vi "Load_Source_Type.vi"(8 "error in (no error)":errorcluster, 9 "index":i32, 11 "buildObject":T1) -> (0 "error out":errorcluster, 3 "AB_Source out":refnum<class "AB_Source.lvclass">)   [LabVIEW 2020, in "AB_Source.lvclass"]
uses:
  <vilib>/AppBuilder/AB_Classes/Source/AB_Source.lvclass
  <resource>/Framework/Providers/API/ItemRef.ctl
  <vilib>/AppBuilder/AB_Classes/Source/VI/AB_Source_VI.lvclass
  e:/builds/penguin/labview/branches/2020/dev/dist/vi.lib/AppBuilder/AB_Classes/Source/AB_Source.lvclass
  <vilib>/AppBuilder/AB_Classes/Source/ExportedVI/AB_Source_ExportedVI.lvclass
  <vilib>/AppBuilder/AB_Classes/Source/RESTfulVI/AB_Source_RESTfulVI.lvclass
  <vilib>/AppBuilder/AB_Classes/Source/Container/AB_Source_Container.lvclass
  <vilib>/AppBuilder/AB_Classes/Source/Library/AB_Source_Library.lvclass
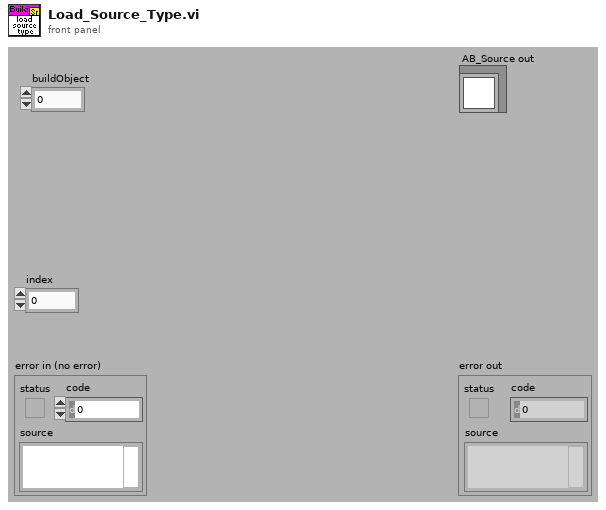
[diagram p1: front panel]
types:
  T1 = typedef "ItemRef.ctl" = u64
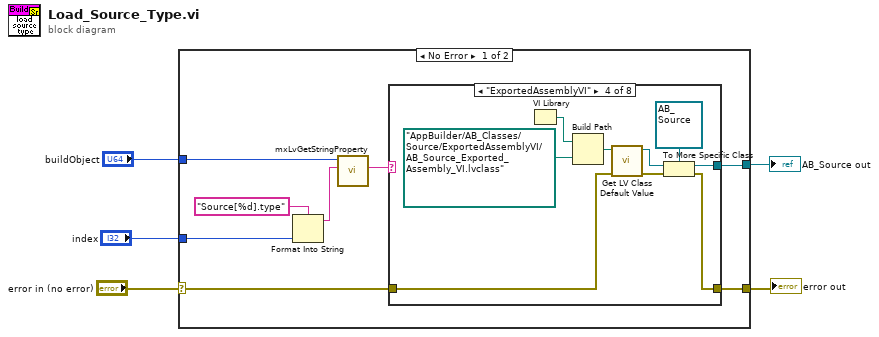
[diagram p0: block diagram]
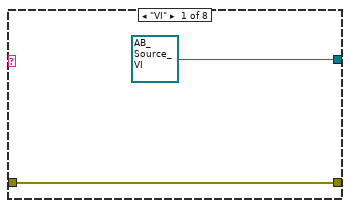
[diagram p2: hidden frame]
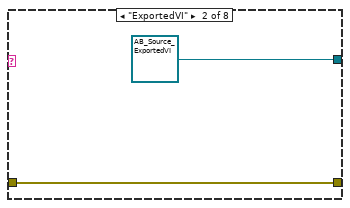
[diagram p3: hidden frame]
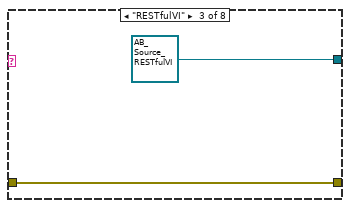
[diagram p4: hidden frame]
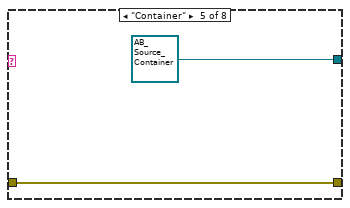
[diagram p5: hidden frame]
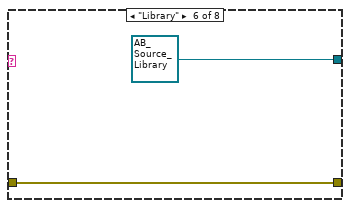
[diagram p6: hidden frame]
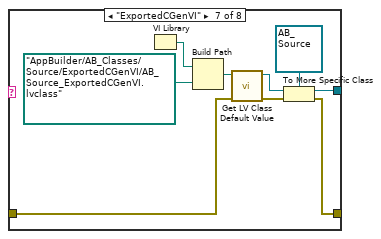
[diagram p7: hidden frame]
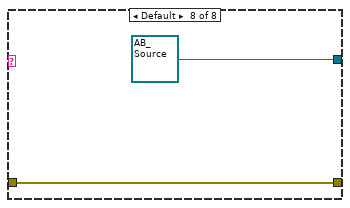
[diagram p8: hidden frame]
diagram:
  n1 = case shown="No Error" "error in (no error)" {
    selector: "error in (no error)" -> [w7 w44]
    tunnel: [w6 w44] -> w4
    tunnel: [w8 _] -> w3
    tunnel: "buildObject" -> [w13 _]
    tunnel: "index" -> [w10 _]
    frame No Error {
      n2 = Format Into String(format string="Source[%d].type", w10) -> (resulting string=w11:string)  [unwired: 2 in, 1 out]
      n3 = call <resource>:"mxLvGetStringProperty.vi"("Tag"=w11, "Item"=w13) -> ("Value"=w9:string)  [unwired: 1 in, 8 out]
      n4 = case shown="\"ExportedAssemblyVI\"" w9 {
        tunnel: [refnum<class "AB_Source_VI.lvclass"> refnum ("AB_Source_VI.lvclass") refnum<class "AB_Source_ExportedVI.lvclass"> refnum ("AB_Source_ExportedVI.lvclass") refnum<class "AB_Source_RESTfulVI.lvclass"> refnum ("AB_Source_RESTfulVI.lvclass") w22 refnum<class "AB_Source_Container.lvclass"> refnum ("AB_Source_Container.lvclass") refnum<class "AB_Source_Library.lvclass"> refnum ("AB_Source_Library.lvclass") w39 refnum<class "AB_Source.lvclass"> refnum ("AB_Source in")] -> w8
        tunnel: w7 -> [w14 w16 w18 w21 w29 w31 w35 w42]
        tunnel: [w14 w16 w18 w20 w29 w31 w33 w42] -> w6
        frame "VI" {
        }
        frame "ExportedVI" {
        }
        frame "RESTfulVI" {
        }
        frame "ExportedAssemblyVI" {
          n5 = VI Library() -> (path=w25:path)
          n6 = Build Path(base path=w25, name or relative path=path "AppBuilder/AB_Classes/Source/ExportedAssemblyVI/AB_Source_Exported_Assembly_VI.lvclass") -> (appended path=w27:path)
          n7 = call <vilib>:"Get LV Class Default Value.vi"("error in (no error)"=w21, "class path"=w27) -> ("error out"=w28:errorcluster, "object"=w24:refnum<class>)  [unwired: 8 in]
          n8 = To More Specific Class(target class=refnum<class "AB_Source.lvclass"> refnum ("AB_Source in"), reference=w24, error in=w28) -> (specific class reference=w22:refnum<class "AB_Source.lvclass">, error out=w20:errorcluster)
        }
        frame "Container" {
        }
        frame "Library" {
        }
        frame "ExportedCGenVI" {
          n9 = VI Library() -> (path=w38:path)
          n10 = Build Path(base path=w38, name or relative path=path "AppBuilder/AB_Classes/Source/ExportedCGenVI/AB_Source_ExportedCGenVI.lvclass") -> (appended path=w36:path)
          n11 = call <vilib>:"Get LV Class Default Value.vi"("error in (no error)"=w35, "class path"=w36) -> ("error out"=w34:errorcluster, "object"=w40:refnum<class>)  [unwired: 8 in]
          n12 = To More Specific Class(target class=refnum<class "AB_Source.lvclass"> refnum ("AB_Source out"), reference=w40, error in=w34) -> (specific class reference=w39:refnum<class "AB_Source.lvclass">, error out=w33:errorcluster)
        }
        frame Default {
        }
      }
    }
    frame Error {
    }
  }
  "error out" <- w4
  "AB_Source out" <- w3
